vi "Edit Instruments Steps.vi"(4 "Adress by Reference?":bool, 5 "Configuration":variant, 6 "Instruments Steps Refnum":refnum<vi>, 7 "error in (no error)":errorcluster, 8 "Instrument":T3=enum."Switching Matrix", 9 "Action":T2, 10 "Instrument Steps In":T1) -> (0 "error out":errorcluster, 3 "Instrument Steps Out":T1)   [LabVIEW 2014]
uses:
  Action.ctl
  Instrument List.ctl
  Instrument Steps.ctl
panel:
  # "LICENSED MATERIALS – PROPERTY OF IBM\nCopyright IBM Corp. 2016,\nALL RIGHTS RESERVED"
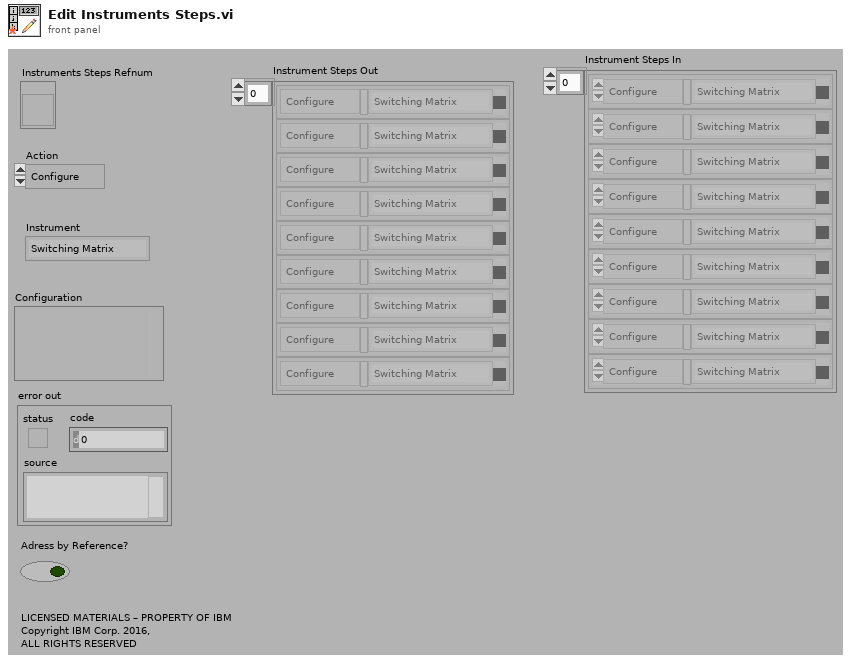
[diagram p1: front panel]
types:
  T1 = typedef "Instrument Steps.ctl" = cluster{"Action":T2, "Configuration":variant, "Instrument":T3, "Status":enum8{"False", "True", "Mixed"}}[]
  T2 = typedef "Action.ctl" = enum32{"Configure", "Measure"}
  T3 = typedef "Instrument List.ctl" = enum32{"Unknown Instrument", "Switching Matrix", "Parameter Analyzer", "Optical Spectrometer", "Optoelectronic", "Autofocus"}
  T4 = cluster{"Action":T2, "Configuration":variant, "Instrument":T3, "Status":enum8{"False", "True", "Mixed"}}
  T5 = cluster{"Action":T2, "Configuration":variant, "Instrument":T3, "Status":enum8{"False", "True", "Mixed"}}[]
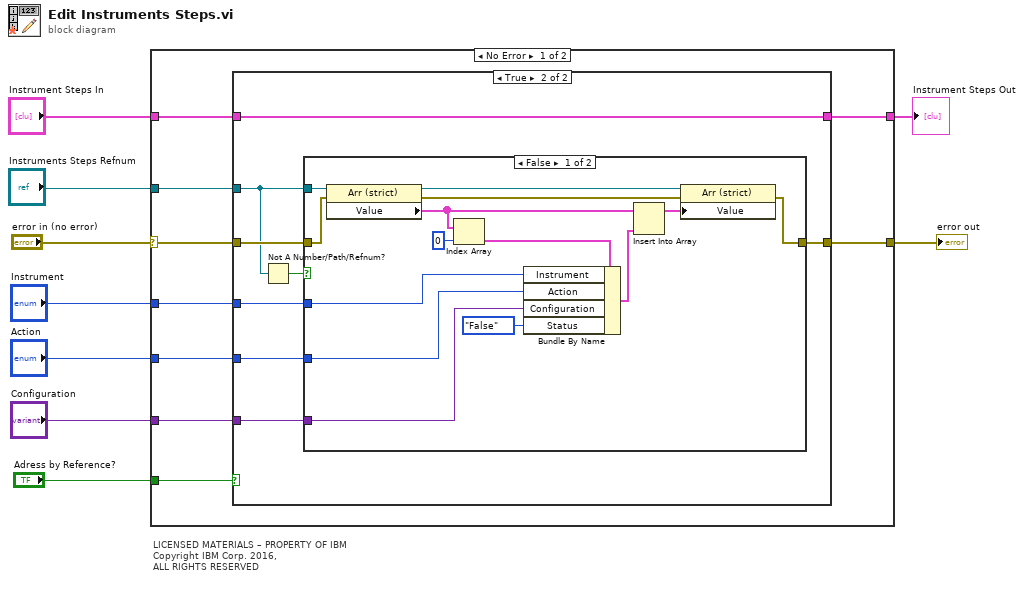
[diagram p0: block diagram]
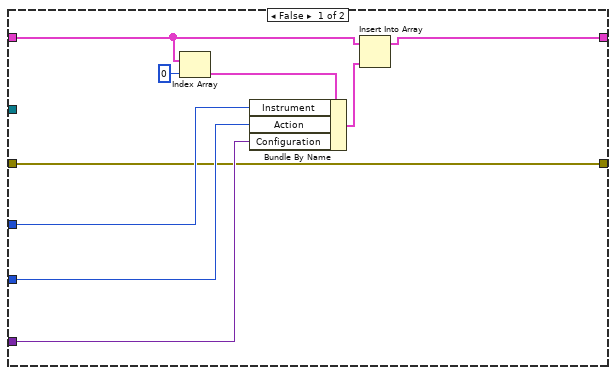
[diagram p2: hidden frame]
diagram:
  # "LICENSED MATERIALS – PROPERTY OF IBM\nCopyright IBM Corp. 2016,\nALL RIGHTS RESERVED"
  n1 = case shown="No Error" "error in (no error)" {
    selector: "error in (no error)" -> [w14 w52]
    tunnel: "Configuration" -> [w18 _]
    tunnel: "Action" -> [w17 _]
    tunnel: "Instrument" -> [w16 _]
    tunnel: "Instruments Steps Refnum" -> [w15 _]
    tunnel: [w13 w52] -> w5
    tunnel: "Adress by Reference?" -> [w12 _]
    tunnel: [w11 w51] -> w2
    tunnel: "Instrument Steps In" -> [w10 w51]
    frame No Error {
      n2 = case shown="True" w12 {
        tunnel: w18 -> [w20 w34]
        tunnel: w17 -> [w21 w33]
        tunnel: w16 -> [w22 w32]
        tunnel: w15 -> [_ w29]
        tunnel: w14 -> [w19 w31]
        tunnel: [w19 w30] -> w13
        tunnel: [w23 w28] -> w11
        tunnel: w10 -> [w24 w28]
        frame False {
          n3 = Index Array(array=w24, index=0) -> (element=w25:T4)
          n4 = Bundle By Name(cluster=w25, "Instrument"=w22, "Action"=w21, "Configuration"=w20) -> (w27:T4)
          n5 = Insert Into Array(array=w24, new element=w27) -> (w23:T1)  [unwired: 1 in]
        }
        frame True {
          n6 = Not A Number/Path/Refnum?(number/path/refnum=w29) -> (NaN/Path/Refnum?=w35:bool)
          n7 = case shown="False" w35 {
            tunnel: w29 -> [w49 _]
            tunnel: w33 -> [w41 _]
            tunnel: w32 -> [w42 _]
            tunnel: w34 -> [w43 _]
            tunnel: w31 -> [w40 w50]
            tunnel: [w38 w50] -> w30
            frame False {
              n8 = property class="Arr (strict)"(reference=w49, error in=w40) -> (reference out=w46:refnum<vi>, error out=w39:errorcluster, "Value"=w45:T5)
              n9 = Index Array(array=w45, index=0) -> (element=w44:T4)
              n10 = Bundle By Name(cluster=w44, "Instrument"=w42, "Action"=w41, "Configuration"=w43, "Status"=enum8{"False", "True", "Mixed"}."False") -> (w48:T4)
              n11 = Insert Into Array(array=w45, new element=w48) -> (w37:T5)  [unwired: 1 in]
              n12 = property class="Arr (strict)"(reference=w46, error in=w39, "Value"=w37) -> (error out=w38:errorcluster)  [unwired: 1 out]
            }
            frame True {
            }
          }
        }
      }
    }
    frame Error {
    }
  }
  "error out" <- w5
  "Instrument Steps Out" <- w2
